vi "Create Event References and Registrations.vi"(8 "error in (no error)":errorcluster) -> (0 "error out":errorcluster, 1 "Event-Registrations":T1, 3 "Event-References":T2)   [LabVIEW 2018, in "Copy of Actor.lvclass"]
uses:
  Copy of Actor.lvclass
  Event-References.ctl
  Stop.ctl
  Launched.ctl
  Some Request.ctl
  Some Response.ctl
  Event-Registrations.ctl
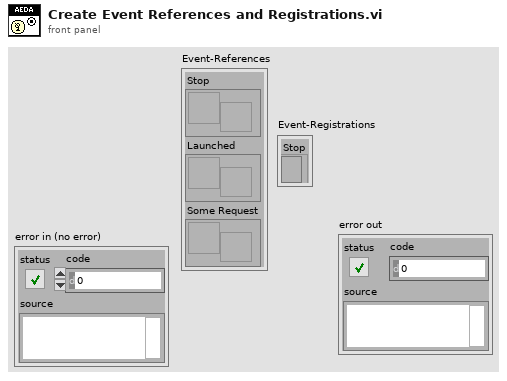
[diagram p1: front panel]
types:
  T1 = typedef "Copy of Actor.lvclass/Event-Registrations.ctl" = cluster{"Stop":refnum<event-registration>}
  T2 = typedef "Copy of Actor.lvclass/Event-References.ctl" = cluster{"Stop":refnum<user-event>, "Launched":refnum<user-event>, "Some Request":refnum<user-event>}
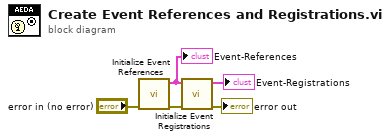
[diagram p0: block diagram]
diagram:
  n1 = call "Initialize Event References.vi"("error in (no error)"="error in (no error)") -> ("error out"=w4:errorcluster, "Event-References"=w3:T2)  [unwired: 9 in]
  "Event-References" <- w3
  n2 = call "Initialize Event Registrations.vi"("error in (no error)"=w4, "Events-References"=w3) -> ("error out"=→"error out":errorcluster, "Event-Registrations"=→"Event-Registrations":T1)  [unwired: 8 in]
